vi "Read DAQmxTasks.vi"(8 "error in":errorcluster, 11 "PAS in":refnum<class "PAS.lvclass">) -> (0 "error out":errorcluster, 2 "DAQmxTasks":T1, 3 "PAS out":refnum<class "PAS.lvclass">)   [LabVIEW 2014, in "PAS.lvclass"]
uses:
  PAS.lvclass
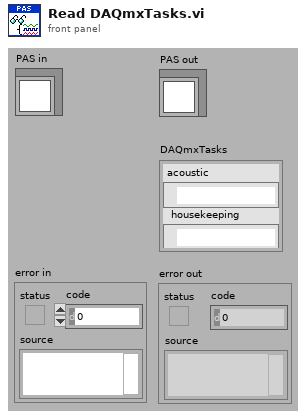
[diagram p1: front panel]
types:
  T1 = cluster{"acoustic":refnum<k21>, "housekeeping":refnum<k21>}
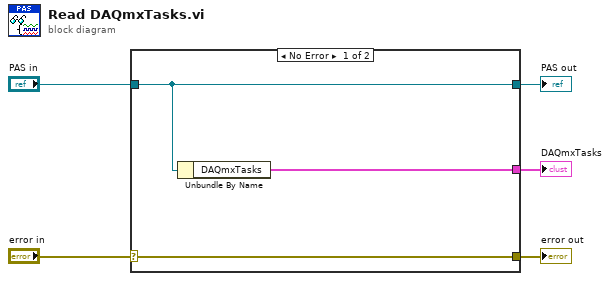
[diagram p0: block diagram]
diagram:
  n1 = case shown="No Error" "error in" {
    selector: "error in" -> [w8 w9]
    tunnel: [w8 w9] -> w4
    tunnel: [w7 w10] -> w2
    tunnel: "PAS in" -> [w7 w10]
    tunnel: [w6 _] -> w1
    frame No Error {
      n2 = Unbundle By Name(w7) -> ("DAQmxTasks"=w6:T1)
    }
    frame Error {
    }
  }
  "error out" <- w4
  "PAS out" <- w2
  "DAQmxTasks" <- w1
